vi "task_2.vi"() -> ()   [LabVIEW 2020]
panel:
  in  "Enter your name":string
  out "Top 3":cluster{"Player1":string, "Score":i32}[](array[cluster])
  out "Player Info":cluster{"Player1":string, "Score":i32}
  in  "Blue":bool
  out "Blue LED":bool
  in  "Red":bool
  out "Red LED":bool
  in  "Green":bool
  out "Green LED":bool
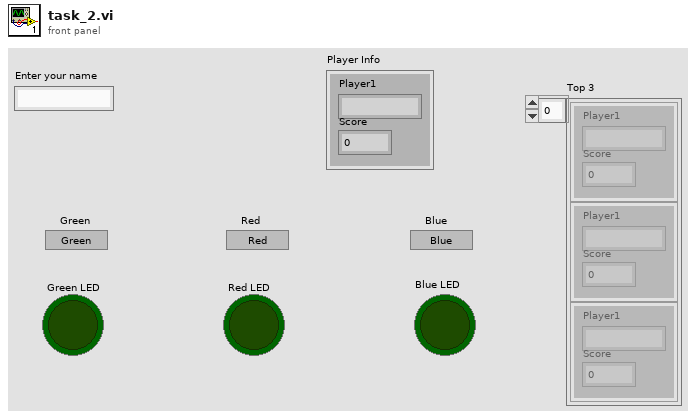
[diagram p1: front panel]
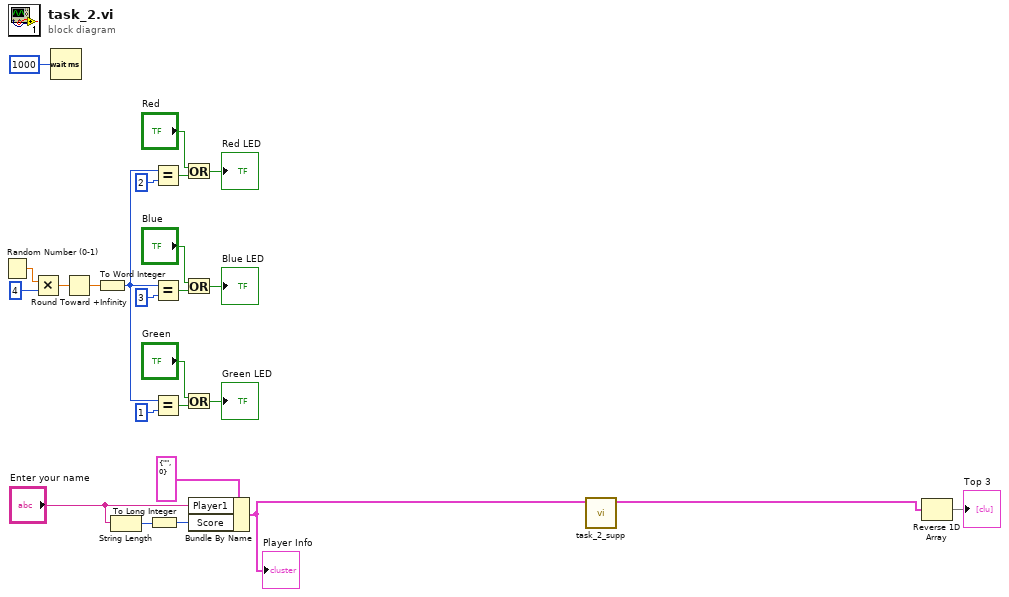
[diagram p0: block diagram]
diagram:
  n1 = Random Number (0-1)() -> (number: 0 to 1=w25:dbl)
  n2 = Multiply(x=w25, y=4) -> (x*y=w24:dbl)
  n3 = Wait (ms)(milliseconds to wait=1000) -> ()  [unwired: 1 out]
  n4 = Round Toward +Infinity(x=w24) -> (ceil(x): smallest int >= x=w22:dbl)
  n5 = To Word Integer(number=w22) -> (16bit integer=w12:i16)
  n6 = String Length(string="Enter your name") -> (length=w8:i32)
  n7 = To Long Integer(number=w8) -> (32bit integer=w5:i32)
  n8 = Equal?(x=w12, y=2) -> (x = y?=w16:bool)
  n9 = Equal?(x=w12, y=3) -> (x = y?=w18:bool)
  n10 = Equal?(x=w12, y=1) -> (x = y?=w21:bool)
  n11 = Or(x="Red", y=w16) -> (x .or. y?=→"Red LED":bool)
  n12 = Or(x="Blue", y=w18) -> (x .or. y?=→"Blue LED":bool)
  n13 = Or(x="Green", y=w21) -> (x .or. y?=→"Green LED":bool)
  n14 = Bundle By Name(cluster=cluster{"Player1":string, "Score":i32} {"Player1"="", "Score"=0} ("Player Info"), "Player1"="Enter your name", "Score"=w5) -> (w2:cluster{"Player1":string, "Score":i32})
  "Player Info" <- w2
  n15 = call "task_2_supp.vi"("Player Info"=w2) -> ("Array"=w1:cluster{"Player1":string, "Score":i32}[])  [unwired: 10 in]
  n16 = Reverse 1D Array(array=w1) -> (reversed array=→"Top 3":cluster{"Player1":string, "Score":i32}[])
